vi "Periodic Tasks.vi"(8 "error in":errorcluster) -> ()   [LabVIEW 2017]
doc: "This VI runs in parallel to other tasks. It can contain as many user-defined periodic loops as you need. These can carry out PID or other sorts of timed response."
uses:
  <vilib>/Rock Robotics/WPI/ThirdParty/Phoenix-LabVIEW/Motor Controller/Controls/CTRE_Phoenix_MotorControl_ControlMode.ctl
  <vilib>/Rock Robotics/WPI/Utilities/WPI_GetSetVariantRefNum.vi
  <vilib>/Rock Robotics/Network Tables/NT Write Boolean.vi
panel:
  out "Distance":dbl
  in  "mode":bool
  out "Waveform Chart":dbl(graph)
  out "current (A)":dbl
  out "Auto Limit?":bool
  out "Motor Setpoint":dbl
  out "Auto Setpoint":dbl
  out "Bottom Limit":bool
  out "Top Limit":bool
  in  "Autonomous":bool
  out "Elevator Speed":dbl
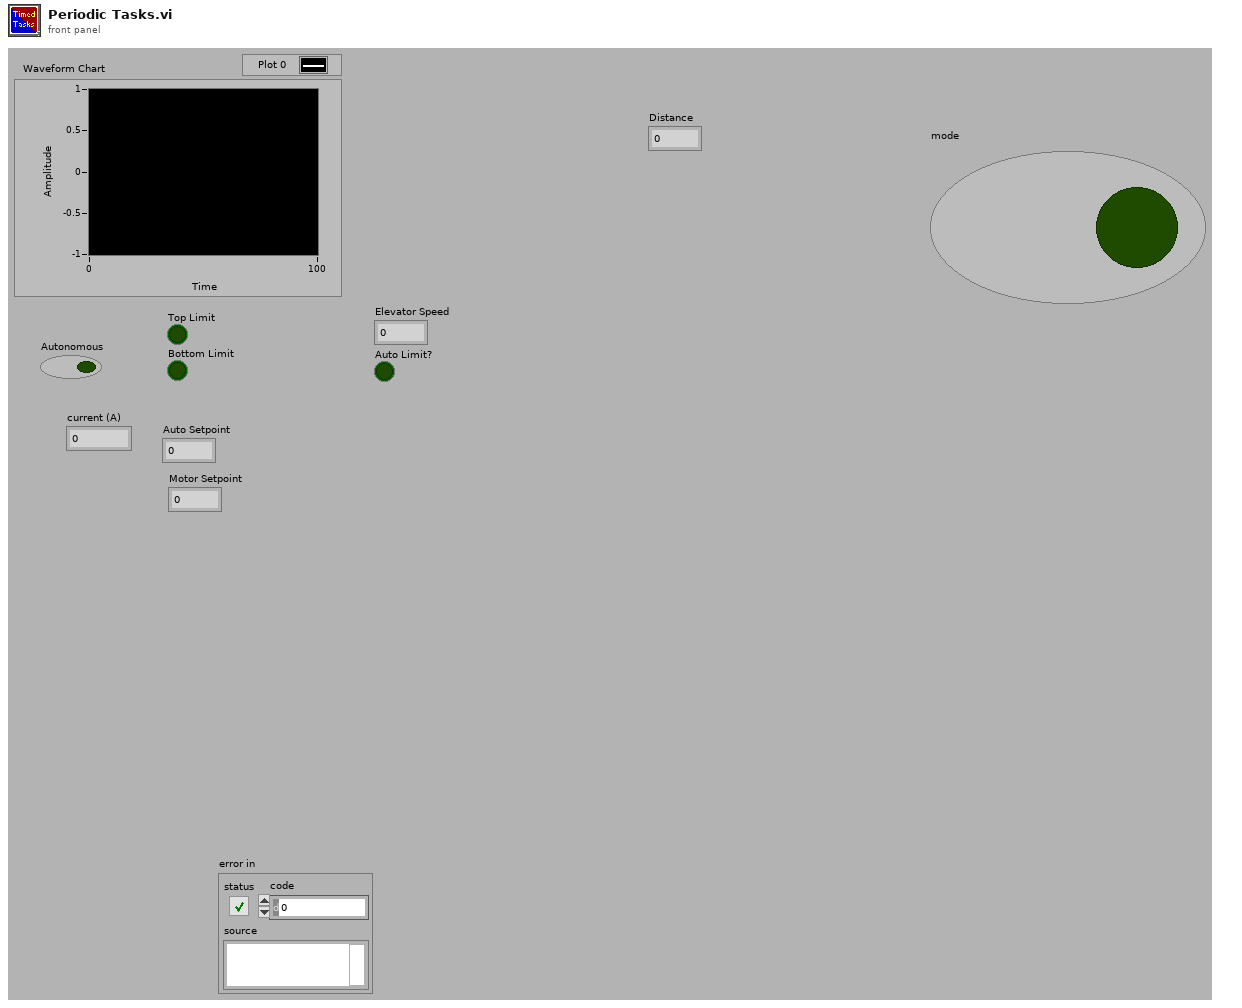
[diagram p1: front panel]
types:
  T1 = enum16{"At limit", "Case1", "Case2", "home", "Init", "Move to home"}
  T2 = typedef "WPI_JoystickDevRef.ctl" = cluster{"Device":T3}
  T3 = typedef "WPI_JoystickDeviceEnum.ctl" = enum16{"USB 0", "USB 1", "USB 2", "USB 3", "USB 4", "USB 5"}
  T4 = typedef "WPI_SwitchDevRef.ctl" = cluster{"DevStatus":errorcluster, "DIO Channel":T5, "CntIndex":T6, "Normally Closed":bool}
  T5 = typedef "FPGA_DIOChannel.ctl" = enum8{"DIO 0", "DIO 1", "DIO 2", "DIO 3", "DIO 4", "DIO 5", "DIO 6", "DIO 7", "DIO 8", "DIO 9", "DIO MXP 0", "DIO MXP 1", "DIO MXP 2", "DIO MXP 3", "DIO MXP 4", "DIO MXP 5", "DIO MXP 6", "DIO MXP 7", "DIO MXP 8", "DIO MXP 9", "DIO MXP 10", "DIO MXP 11", "DIO MXP 12", "DIO MXP 13", "DIO MXP 14", "DIO MXP 15", "SPI Port CS1", "SPI Port CS2", "SPI Port CS3", "SPI Port MISO", "SPI Port MOSI", "Invalid"}
  T6 = typedef "FPGA_CounterCtrSystemIndex.ctl" = enum8{"Ctr 0", "Ctr 1", "Ctr 2", "Ctr 3", "Ctr 4", "Ctr 5", "Ctr 6", "Ctr 7", "Invalid"}
  T7 = typedef "WPI_MotorControlDeviceRef.ctl" = cluster{"DeviceStatus":errorcluster, "Type":T8, "PWM":cluster{"PWM Channel":T9, "DeadBand":T10}, "CAN":cluster{"Device Number":u8, "SetOutput VI Ref":variant, "GetOutput VI Ref":variant, "Enable VI Ref":variant, "Disable VI Ref":variant, "Data":variant}, "Invert":bool, "DIO PWM":cluster{"PWM \"Enable\" Channel":T9, "DIOChannel":T5, "PWM Rate":dbl}}
  T8 = typedef "WPI_MotorControlType.ctl" = enum16{"PWM", "CAN", "DIO PWM"}
  T9 = typedef "FPGA_DIOPWMChannel.ctl" = enum8{"PWM 0", "PWM 1", "PWM 2", "PWM 3", "PWM 4", "PWM 5", "PWM 6", "PWM 7", "PWM 8", "PWM 9", "PWM MXP 0", "PWM MXP 1", "PWM MXP 2", "PWM MXP 3", "PWM MXP 4", "PWM MXP 5", "PWM MXP 6", "PWM MXP 7", "PWM MXP 8", "PWM MXP 9", "Invalid"}
  T10 = typedef "WPI_PWMDeadband.ctl" = cluster{"Name":string, "maxPositivePwm":i32, "minPositivePwm":i32, "centerPwm":i32, "maxNegativePwm":i32, "minNegativePwm":i32, "angularRange":u16}
  T11 = enum16{"At limit", "Case1", "Case2", "home", "Init"}
  T12 = typedef "CTRE_Phoenix_MotorControl_ControlMode.ctl" = u16
  T13 = typedef "WPI_EncoderDevRef.ctl" = cluster{"DevStatus":errorcluster, "EncoderIndex":T14, "CounterIndex":T6, "DistancePerCount":dbl, "Decoding Type":T15}
  T14 = typedef "FPGA_EncoderIdx.ctl" = enum8{"Enc 0", "Enc 1", "Enc 2", "Enc 3", "Enc 4", "Enc 5", "Enc 6", "Enc 7", "Invalid"}
  T15 = typedef "WPI_EncoderType.ctl" = enum16{"1x", "2x", "4x"}
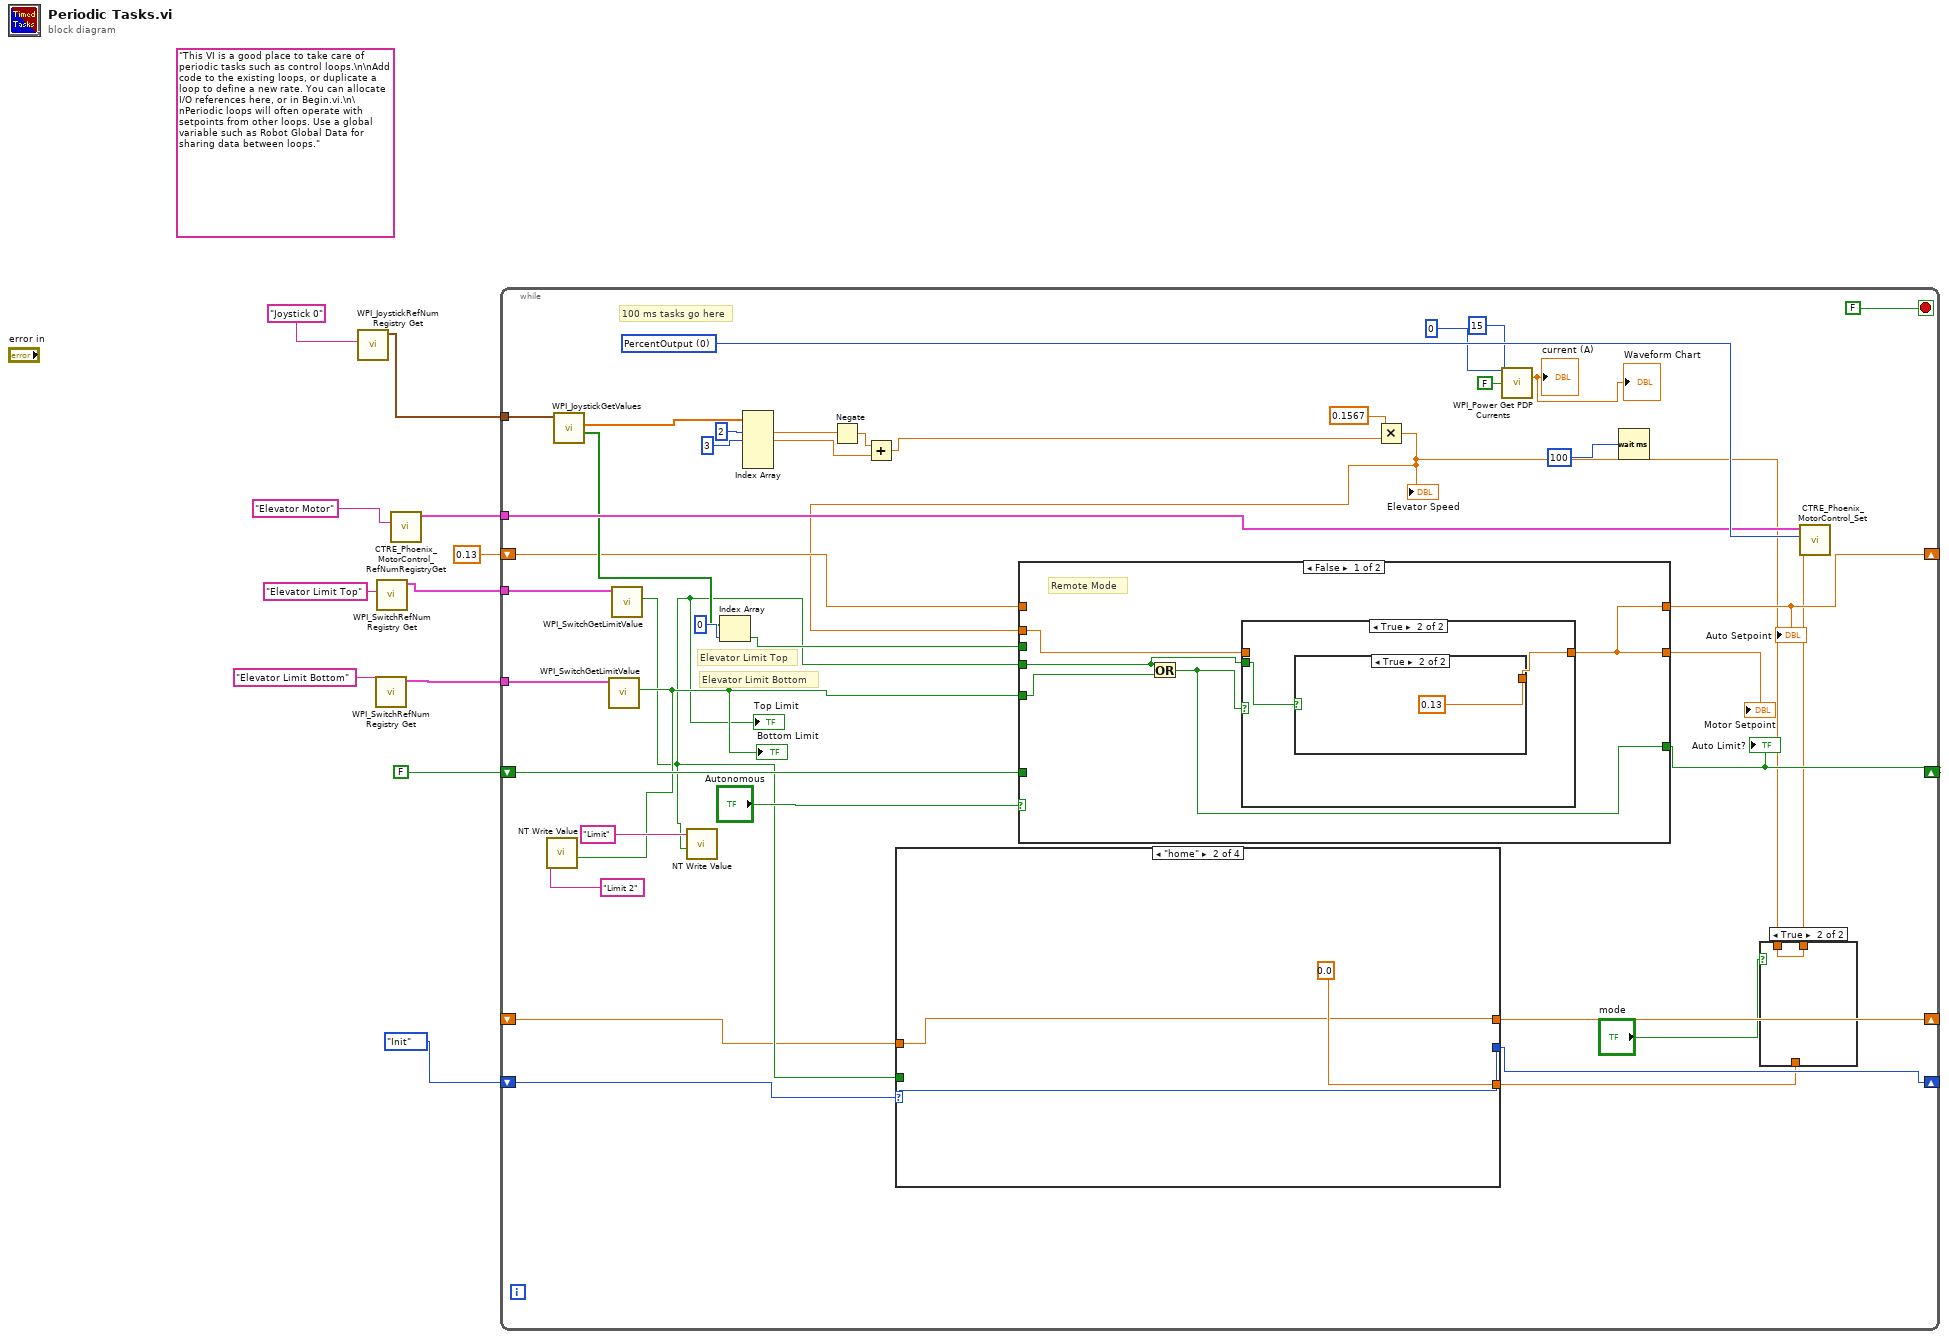
[diagram p0: block diagram]
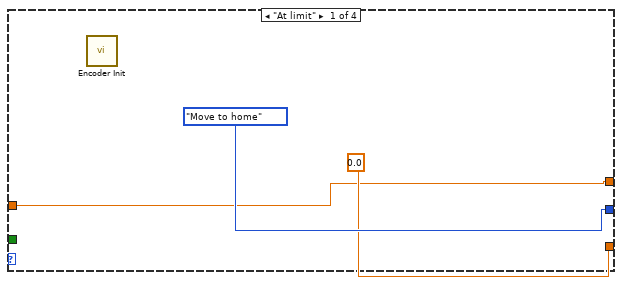
[diagram p3: hidden frame]
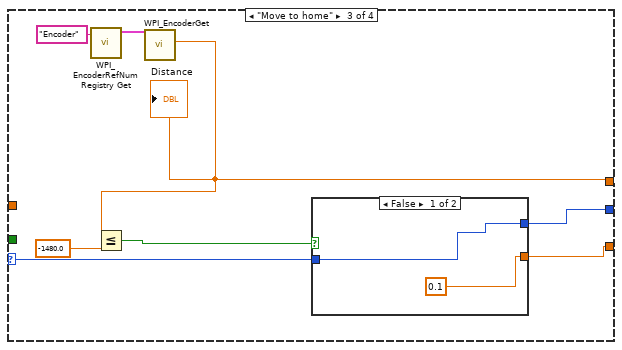
[diagram p4: hidden frame]
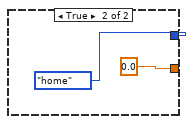
[diagram p5: hidden frame]
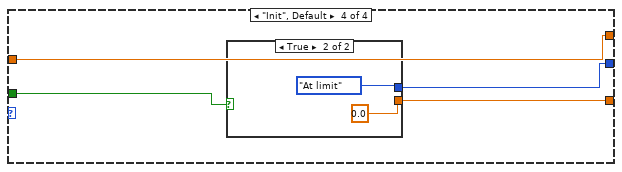
[diagram p6: hidden frame]
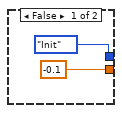
[diagram p7: hidden frame]
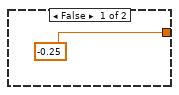
[diagram p9: hidden frame]
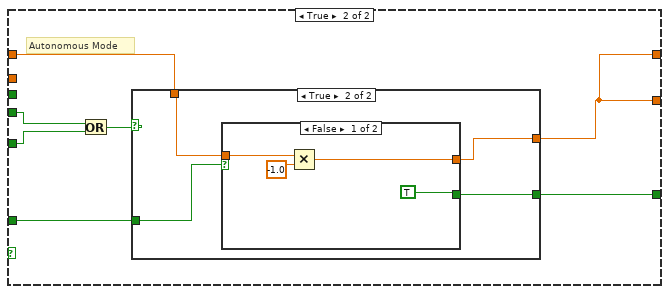
[diagram p10: hidden frame]
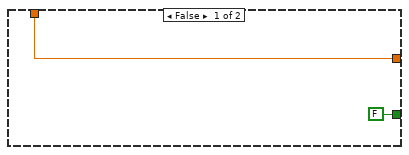
[diagram p11: hidden frame]
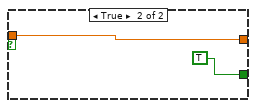
[diagram p12: hidden frame]
diagram:
  (unwired) "This VI is a good place to take care of periodic tasks such as control loops.\n\nAdd code to the existing loops, or duplicate a loop to define a new rate. You can allocate I/O references here, or in Begin.vi.\n\nPeriodic loops will often operate with setpoints from other loops. Use a global variable such as Robot Global Data for sharing data between loops."
  n1 = call <vilib>:"WPI_JoystickRefNum Registry Get.vi"("refnum name"="Joystick 0") -> ("JoystickDevRef"=w4:T2)  [unwired: 1 in, 9 out]
  n2 = call <vilib>:"WPI_SwitchRefNum Registry Get.vi"("refnum name"="Elevator Limit Bottom") -> ("SwitchDevRef"=w7:T4)  [unwired: 9 in, 1 out]
  n3 = call <vilib>:"WPI_SwitchRefNum Registry Get.vi"("refnum name"="Elevator Limit Top") -> ("SwitchDevRef"=w6:T4)  [unwired: 9 in, 1 out]
  n4 = call <vilib>:"CTRE_Phoenix_MotorControl_RefNumRegistryGet.vi"("refnum name"="Elevator Motor") -> ("PhoenixMotorControlDevRef"=w5:T7)  [unwired: 9 in, 1 out]
  n5 = while {
    tunnel: w7 -> [w39]
    tunnel: w6 -> [w38]
    tunnel: w5 -> [w37]
    tunnel: w4 -> [w36]
    shift-right: [w20] -> _
    shift-left: 0.13 -> [w31]
    shift-right: [w29] -> _
    shift-left: FALSE ("Limit State") -> [w30]
    shift-right: [w18] -> _
    shift-left: T1."Init" -> [w19]
    shift-right: [w17] -> _
    shift-left: _ -> [w12]
    stop <- FALSE stop-if-true
    w48 = T12 0 items=["PercentOutput"=0, "Position"=1, "Velocity"=2, "Current"=3, "Follower"=5, "MotionProfile"=6, "MotionMagic"=7, "MotionMagicArc"=8, "MotionProfileArc"=10, "Disabled"=15] ("Control Mode")
    # "Elevator Limit Bottom"
    # "Elevator Limit Top"
    # "100 ms tasks go here"
    n6 = call <vilib>:"WPI_JoystickGetValues.vi"("JoystickDevRef"=w36) -> ("Buttons"=w33:bool[], "Axes"=w49:dbl[])  [unwired: 6 in, 3 out]
    n7 = call <vilib>:"WPI_SwitchGetLimitValue.vi"("SwitchDevRef"=w39) -> ("Switch Pressed"=w28:bool)  [unwired: 8 in, 2 out]
    "Bottom Limit" <- w28
    n8 = call-poly <vilib>:"NT Write Value.vi"("Boolean"=w28, "Name"="Limit 2") -> ()  [unwired: 9 in, 1 out]
    n9 = call <vilib>:"WPI_SwitchGetLimitValue.vi"("SwitchDevRef"=w38) -> ("Switch Pressed"=w21:bool)  [unwired: 8 in, 2 out]
    "Top Limit" <- w21
    n10 = call-poly <vilib>:"NT Write Value.vi"("Boolean"=w21, "Name"="Limit") -> ()  [unwired: 9 in, 1 out]
    n11 = Index Array(array=w33, index=0) -> (element=w32:bool)
    n12 = Index Array(array=w49, index #1=2 ("index"), index #2=3 ("index")) -> (element #1=w41:dbl, element #2=w42:dbl)  [unwired: 3 in, 3 out]
    n13 = Negate(x=w41) -> (-x=w40:dbl)
    n14 = Add(x=w40, y=w42) -> (x+y=w22:dbl)
    n15 = case shown="\"home\"" w19 {
      selector: w19 -> [_ w58 w64 _]
      tunnel: w21 -> [_ _ _ w75]
      tunnel: [T1."Move to home" w58 w67 w73] -> w18
      tunnel: [0.0 0.0 w65 w74] -> w16
      tunnel: [w54 w57 w60 w72] -> w17
      tunnel: w12 -> [w54 w57 _ w72]
      frame "At limit" {
        n16 = call "Encoder Init.vi"() -> ()  [unwired: 12 in]
      }
      frame "home" {
      }
      frame "Move to home" {
        n17 = call <vilib>:"WPI_EncoderRefNum Registry Get.vi"("refnum name"="Encoder") -> ("EncoderDevRef"=w61:T13)  [unwired: 9 in, 1 out]
        n18 = call <vilib>:"WPI_EncoderGet.vi"("EncoderDevRef"=w61) -> ("Distance"=w60:dbl)  [unwired: 5 in, 5 out]
        "Distance" <- w60
        n19 = Less Or Equal?(x=w60, y=-1480.0) -> (x <= y?=w66:bool)
        n20 = case shown="False" w66 {
          tunnel: [w68 T1."home"] -> w67
          tunnel: [0.1 0.0] -> w65
          tunnel: w64 -> [w68 _]
          frame False {
          }
          frame True {
          }
        }
      }
      frame "Init", Default {
        n21 = case shown="True" w75 {
          tunnel: [-0.1 0.0] -> w74
          tunnel: [T11."Init" T11."At limit"] -> w73
          frame False {
          }
          frame True {
          }
        }
      }
    }
    n22 = Multiply(x=0.1567 ("y"), y=w22) -> (x*y=w14:dbl)
    "Elevator Speed" <- w14
    n23 = case shown="False" "Autonomous" {
      tunnel: w32 -> [_ _]
      tunnel: w14 -> [w81 _]
      tunnel: w21 -> [w82 w95]
      tunnel: w28 -> [w84 w96]
      tunnel: [w80 w90] -> w23
      tunnel: w31 -> [_ w93]
      tunnel: [w80 w90] -> w20
      tunnel: w30 -> [_ w92]
      tunnel: [w83 w91] -> w29
      frame False {
        # "Remote Mode"
        n24 = Or(x=w82, y=w84) -> (x .or. y?=w83:bool)
        n25 = case shown="True" w83 {
          tunnel: w81 -> [w85 _]
          tunnel: [w85 w87] -> w80
          tunnel: w82 -> [_ w86]
          frame False {
          }
          frame True {
            n26 = case shown="True" w86 {
              tunnel: [-0.25 0.13] -> w87
              frame False {
              }
              frame True {
              }
            }
          }
        }
      }
      frame True {
        # "Autonomous Mode"
        n27 = Or(x=w95, y=w96) -> (x .or. y?=w94:bool)
        n28 = case shown="True" w94 {
          tunnel: w93 -> [w98 w102]
          tunnel: [w98 w101] -> w90
          tunnel: w92 -> [_ w100]
          tunnel: [FALSE w99] -> w91
          frame False {
          }
          frame True {
            n29 = case shown="False" w100 {
              tunnel: w102 -> [w106 w108]
              tunnel: [w104 w108] -> w101
              tunnel: [TRUE TRUE] -> w99
              frame False {
                n30 = Multiply(x=w106, y=-1.0) -> (x*y=w104:dbl)
              }
              frame True {
              }
            }
          }
        }
      }
    }
    "Auto Setpoint" <- w20
    "Motor Setpoint" <- w23
    "Auto Limit?" <- w29
    n31 = call <vilib>:"WPI_Power Get PDP Currents.vi"("Power Distribution Panel (0)"=u8 0, "PDP Channel"=15, "Tare Currents?"=FALSE) -> ("current (A)"=→"current (A)" →"Waveform Chart":dbl)  [unwired: 10 in, 2 out]
    n32 = Wait (ms)(milliseconds to wait=u32 100) -> ()  [unwired: 1 out]
    n33 = case shown="True" "mode" {
      tunnel: w16 -> [w52 _]
      tunnel: [w52 w53] -> w15
      tunnel: w14 -> [_ w53]
      frame False {
      }
      frame True {
      }
    }
    n34 = call <vilib>:"CTRE_Phoenix_MotorControl_Set.vi"("Output"=w15, "Control Mode"=w48, "PhoenixMotorControlDevRef"=w37) -> ()  [unwired: 7 in, 2 out]
  }
